vi "Set Button From Object.vi"(0 "Display State In":T1={"Buttons Displayed"=0, "Button States"=[], "Button Size"=0, "Button Style"=enum."Classic", "Active Button"=0, "Force Regen?"=FALSE, "Tip String Ref"=refnum}, 5 "Index (-1=at end)":i32=-1, 7 "Insert (F=Replace)":bool, 9 "Container State":T3={"Indicator?"=FALSE, "Run Mode?"=TRUE, " Refnum"=refnum}, 11 "error in (no error)":errorcluster, 12 "Button.lvclass":refnum<class "Button.lvclass">) -> (4 "Display State Out":T1={"Buttons Displayed"=0, "Button States"=[], "Button Size"=0, "Button Style"=enum."Classic", "Active Button"=0, "Force Regen?"=FALSE, "Tip String Ref"=refnum}, 15 "error out":errorcluster)   [LabVIEW 2012, in "Toolbar.xctl"]
doc: "Set the toolbar button state directly from a Button class instance"
uses:
  Toolbar.xctl
  <vilib>/_xctls/Container State.ctl
  Toolbar State.ctl
  Button_Class/Button.lvclass
  Button_Class/Type Defs/Button Style.ctl
  Button_Class/Type Defs/Button Status.ctl
  <vilib>/_xctls/XControlSupport.lvlib
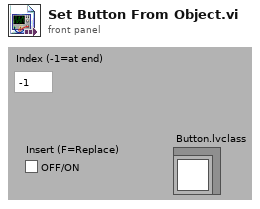
[diagram p1: front panel]
types:
  T1 = typedef "Toolbar.xctl/Toolbar State.ctl" = cluster{"Buttons Displayed":i32, "Button States":refnum<class "Button.lvclass">[], "Button Size":i32, "Button Style":T2, "Active Button":i32, "Force Regen?":bool, "Tip String Ref":refnum<vi>}
  T2 = typedef "Button.lvclass/Button Style.ctl" = enum16{"System", "Modern", "Classic", "Rounded", "Silver", "Ni Theme", "Metallic"}
  T3 = typedef "XControlSupport.lvlib/Container State.ctl" = cluster{"Indicator?":bool, "Run Mode?":bool, " Refnum":refnum<vi>}
  T4 = typedef "Button.lvclass/Button Status.ctl" = enum16{"Off", "Hover", "On", "Disabled"}
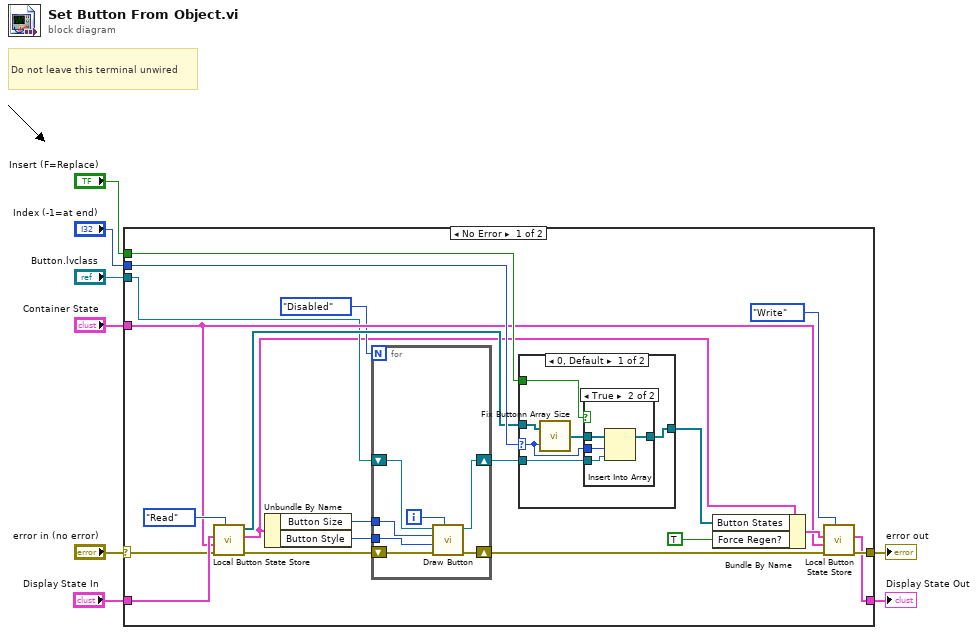
[diagram p0: block diagram]
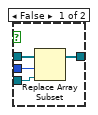
[diagram p2: hidden frame]
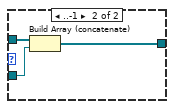
[diagram p3: hidden frame]
diagram:
  # "Do not leave this terminal unwired"
  n1 = case shown="No Error" "error in (no error)" {
    selector: "error in (no error)" -> [w17 w54]
    tunnel: "Display State In" -> [w24 w55]
    tunnel: [w21 w55] -> w7
    tunnel: [w25 w54] -> w6
    tunnel: "Index (-1=at end)" -> [w29 _]
    tunnel: "Button.lvclass" -> [w18 _]
    tunnel: "Insert (F=Replace)" -> [w28 _]
    tunnel: "Container State" -> [w20 _]
    frame No Error {
      n2 = call "Local Button State Store.vi"("Operation"=enum16{"Read", "Write"}."Read", "error in (no error)"=w17, "Container State"=w20, "Display State In"=w24) -> ("error out"=w16:errorcluster, "Display State Out"=w12:T1, "Button States"=w23:refnum<class "Button.lvclass">[])  [unwired: 5 out]
      n3 = Unbundle By Name(w12) -> ("Button Size"=w11:i32, "Button Style"=w10:T2)
      n4 = for {
        N: Button_Status."Disabled" ("Button State") -> [_]
        shift-right: [w35] -> w14
        shift-left: w18 -> [w36]
        shift-right: [w33] -> w15
        shift-left: w16 -> [w34]
        tunnel: w11 -> [w31]
        tunnel: w10 -> [w30]
        i -> [w32]
        n5 = call "Draw Button.vi"("Button State"=w32, "error in (no error)"=w34, "Button Style"=w30, "Button Size"=w31, "Button.lvclass"=w36) -> ("error out"=w33:errorcluster, "Button.lvclass Out"=w35:refnum<class "Button.lvclass">)  [unwired: 1 in, 4 out]
      }
      n6 = case shown="0, Default" w29 {
        selector: w29 -> [w40 _]
        tunnel: w23 -> [w37 w53]
        tunnel: w14 -> [w39 w52]
        tunnel: [w38 w51] -> w9
        tunnel: w28 -> [w42 _]
        frame 0, Default {
          n7 = call "Fix Buttonn Array Size.vi"("Number of Buttons"=w40, "Button States In"=w37) -> ("Button States Out"=w41:refnum<class "Button.lvclass">[])
          n8 = case shown="True" w42 {
            tunnel: w41 -> [w46 w50]
            tunnel: w40 -> [w45 w48]
            tunnel: w39 -> [w44 w49]
            tunnel: [w43 w47] -> w38
            frame False {
              n9 = Replace Array Subset(array=w46, new element=w44, index=w45) -> (w43:refnum<class "Button.lvclass">[])
            }
            frame True {
              n10 = Insert Into Array(array=w50, index=w48, new element=w49) -> (w47:refnum<class "Button.lvclass">[])
            }
          }
        }
        frame ..-1 {
          n11 = Build Array (concatenate)(w53, w52) -> (w51:refnum<class "Button.lvclass">[])
        }
      }
      n12 = Bundle By Name(cluster=w12, "Button States"=w9, "Force Regen?"=TRUE) -> (w22:T1)
      n13 = call "Local Button State Store.vi"("Operation"=enum16{"Read", "Write"}."Write", "error in (no error)"=w15, "Container State"=w20, "Display State In"=w22) -> ("error out"=w25:errorcluster, "Display State Out"=w21:T1)  [unwired: 1 in, 5 out]
    }
    frame Error {
    }
  }
  "Display State Out" <- w7
  "error out" <- w6
